vi "Merge Label String.vi"(4 "Draw Major Tick?":bool, 6 "Draw Major Grid?":bool, 7 "Format String":string, 8 "error in (no error)":errorcluster, 9 "Logarithm?":bool, 10 "Tick Value Array":sgl[](array[numeric]), 11 "Value Pair Cluster":T1) -> (0 "error out":errorcluster, 3 "Tick Cluster Array":T2)   [LabVIEW 2020, in "3D Plot.lvclass"]
uses:
  3D Plot.lvclass
  Tick Array.ctl
  Value Pair Cluster.ctl
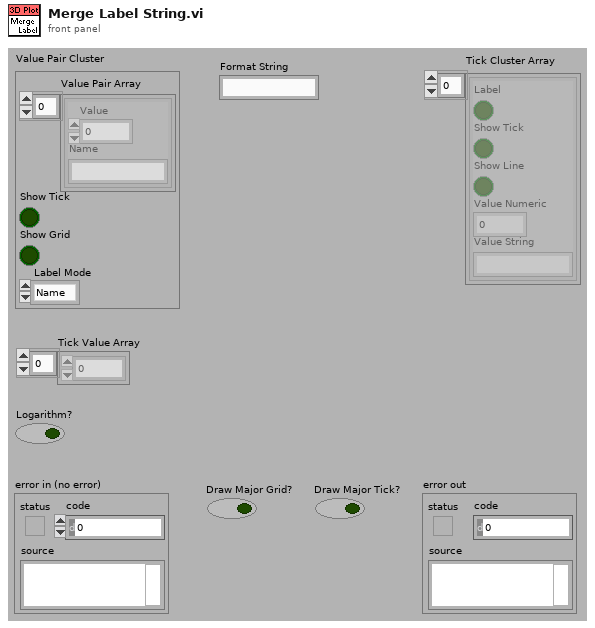
[diagram p1: front panel]
types:
  T1 = typedef "3D Plot.lvclass/Value Pair Cluster.ctl" = cluster{"Value Pair Array":cluster{"Value":sgl, "Name":string}[], "Show Tick":bool, "Show Grid":bool, " Label Mode":enum16{"Name", "Value", "None"}}
  T2 = typedef "3D Plot.lvclass/Tick Array.ctl" = cluster{"Label":bool, "Show Tick":bool, "Show Line":bool, "Value Numeric":sgl, "Value String":string}[]
  T3 = cluster{"Show ticks":bool, "Show ticks":bool, "Show ticks":bool, "Interval":sgl, string}
  T4 = cluster{"Show ticks":bool, "Show ticks":bool, "Show ticks":bool, "Interval":sgl, string}[]
  T5 = cluster{"Show ticks":bool, "Show Tick":bool, "Show Grid":bool, "Value":sgl, "Name":string}
  T6 = cluster{"Show ticks":bool, "Draw Major Tick?":bool, "Draw Major Grid?":bool, "Interval":sgl, string}
  T7 = cluster{"Show ticks":bool, "Show Tick":bool, "Show Grid":bool, "Interval":sgl, "Name":string}
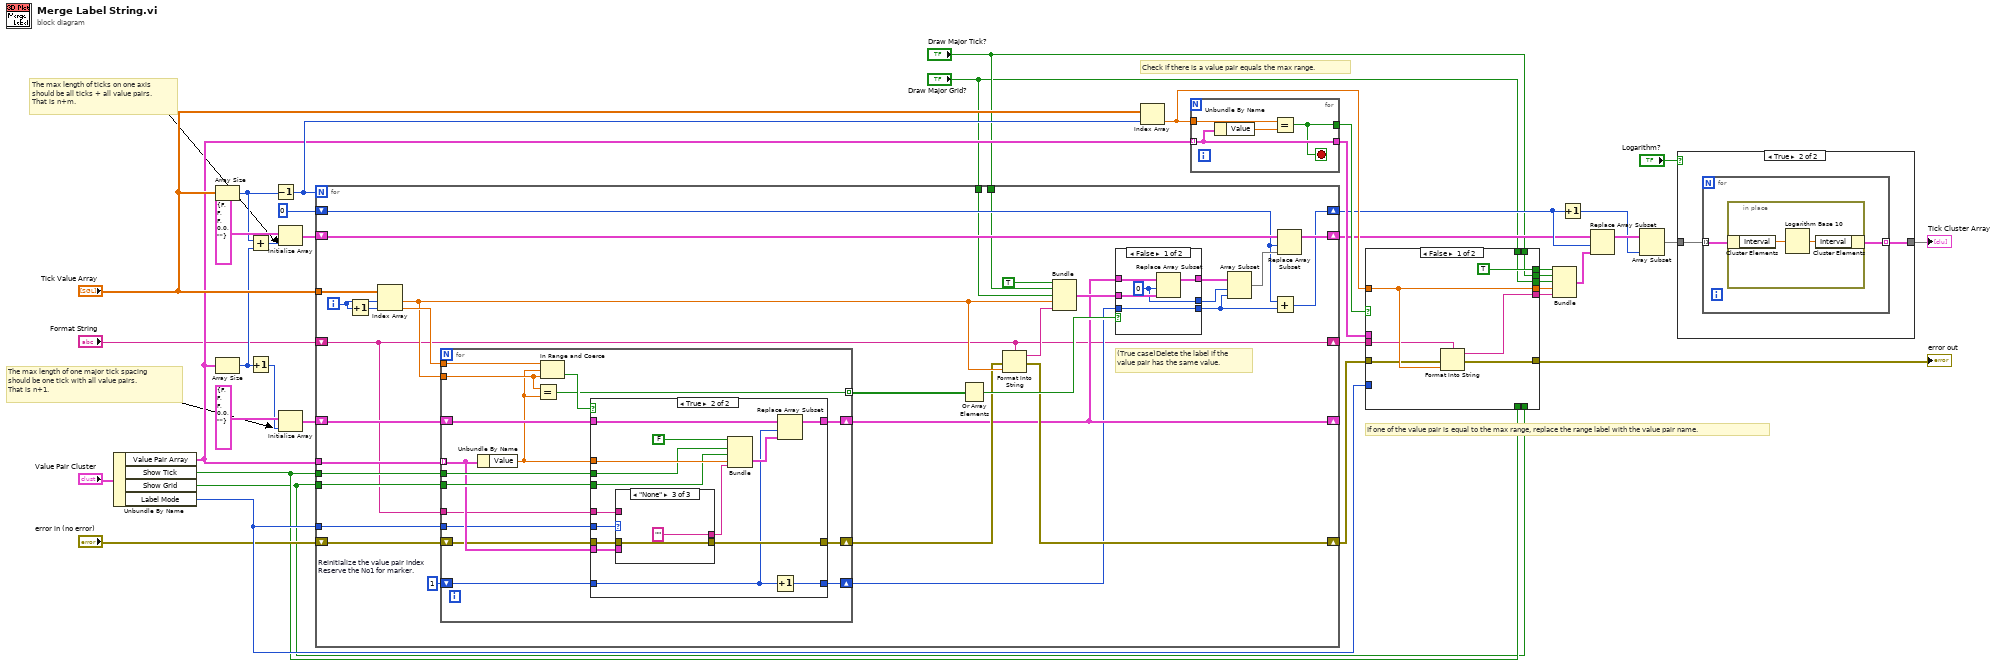
[diagram p0: block diagram]
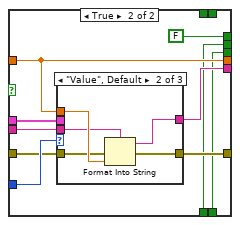
[diagram p3: hidden frame]
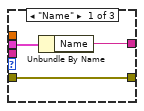
[diagram p4: hidden frame]
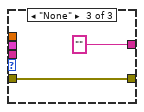
[diagram p5: hidden frame]
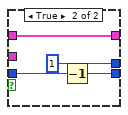
[diagram p6: hidden frame]
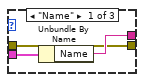
[diagram p8: hidden frame]
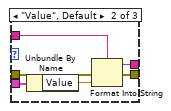
[diagram p9: hidden frame]
diagram:
  # "Check if there is a value pair equals the max range."
  # "The max length of ticks on one axis\nshould be all ticks + all value pairs.\nThat is n+m."
  # "The max length of one major tick spacing \nshould be one tick with all value pairs.\nThat is n+1."
  # "If one of the value pair is equal to the max range, replace the range label with the value pair name."
  n1 = Unbundle By Name("Value Pair Cluster") -> ("Value Pair Array"=w23:cluster{"Value":sgl, "Name":string}[], "Show Tick"=w2:bool, "Show Grid"=w1:bool, "Label Mode"=w34:enum16{"Name", "Value", "None"})
  n2 = Array Size(array="Tick Value Array") -> (size(s)=w19:i32)
  n3 = Array Size(array=w23) -> (size(s)=w18:i32)
  n4 = Add(x=w19, y=w18) -> (x+y=w17:i32)
  n5 = Increment(x=w18) -> (x+1=w22:i32)
  n6 = Decrement(x=w19) -> (x-1=w39:i32)
  n7 = Initialize Array(T3 {"Show ticks"=FALSE, "Show ticks"=FALSE, "Show ticks"=FALSE, "Interval"=0.0, ""}, w17) -> (w20:T4)
  n8 = Initialize Array(T3 {"Show ticks"=FALSE, "Show ticks"=FALSE, "Show ticks"=FALSE, "Interval"=0.0, ""}, w22) -> (w24:T4)
  n9 = for {
    N: w39 -> [_]
    tunnel: "Tick Value Array" -> [w70]
    tunnel: w23 -> [w55]
    tunnel: w2 -> [w64]
    tunnel: w1 -> [w63]
    tunnel: w34 -> [w66]
    shift-right: [w47] -> w10
    shift-left: w20 -> [w48]
    shift-right: [w56] -> w27
    shift-left: "error in (no error)" -> [w58]
    shift-right: [w52] -> _
    shift-left: w24 -> [w53]
    shift-right: [w43] -> w12
    shift-left: 0 -> [w45]
    shift-right: [w42] -> w8
    shift-left: "Format String" -> [w42]
    tunnel: "Draw Major Grid?" -> [w40]
    tunnel: "Draw Major Tick?" -> [w41]
    i -> [w68]
    w54 = 1  # Reinitialize the value pair index Reserve the No1 for marker.
    # "(True case)Delete the label if the \nvalue pair has the same value."
    n10 = Increment(x=w68) -> (x+1=w69:i32)
    n11 = Index Array(array=w70, index #1=w68, index #2=w69) -> (element #1=w60:sgl, element #2=w67:sgl)
    n12 = for {
      tunnel: w55 -> [w88] mode=indexing
      shift-right: [w94] -> w52
      shift-left: w53 -> [w93]
      tunnel: w67 -> [w96]
      tunnel: w60 -> [w89]
      tunnel: w66 -> [w86]
      tunnel: w42 -> [w87]
      tunnel: [w90] -> w62 mode=indexing
      tunnel: w64 -> [w92]
      tunnel: w63 -> [w91]
      shift-right: [w84] -> w57
      shift-left: w58 -> [w83]
      shift-right: [w81] -> w49
      shift-left: w54 -> [w82]
      n13 = Unbundle By Name(w88) -> ("Value"=w85:sgl)
      n14 = Equal?(x=w89, y=w85) -> (x = y?=w90:bool)
      n15 = In Range and Coerce(upper limit=w96, x=w85, lower limit=w89) -> (In Range?=w95:bool)  [unwired: 1 out]
      n16 = case shown="True" w95 {
        tunnel: w85 -> [_ w114]
        tunnel: [w99 w103] -> w94
        tunnel: w93 -> [w99 w104]
        tunnel: w92 -> [_ w112]
        tunnel: w91 -> [_ w111]
        tunnel: w88 -> [_ w110]
        tunnel: w87 -> [_ w109]
        tunnel: w86 -> [_ w108]
        tunnel: [w98 w106] -> w84
        tunnel: w83 -> [w98 w105]
        tunnel: w82 -> [w97 w100]
        tunnel: [w97 w101] -> w81
        frame False {
        }
        frame True {
          n17 = case shown="\"None\"" w108 {
            tunnel: w110 -> [w117 w123 _]
            tunnel: [w116 w120 ""] -> w107
            tunnel: w109 -> [_ w122 _]
            tunnel: [w115 w119 w124] -> w106
            tunnel: w105 -> [w115 w118 w124]
            frame "Name" {
              n18 = Unbundle By Name(w117) -> ("Name"=w116:string)
            }
            frame "Value", Default {
              n19 = Unbundle By Name(w123) -> ("Value"=w121:sgl)
              n20 = Format Into String(format string=w122, error in=w118, w121) -> (resulting string=w120:string, error out=w119:errorcluster)  [unwired: 1 in]
            }
            frame "None" {
            }
          }
          n21 = Bundle("Show ticks"=FALSE, "Show Tick"=w112, "Show Grid"=w111, "Value"=w114, "Name"=w107) -> (w102:T5)  [unwired: 1 out]
          n22 = Increment(x=w100) -> (x+1=w101:i32)
          n23 = Replace Array Subset(array=w104, new element=w102, index=w100) -> (w103:T4)
        }
      }
    }
    n24 = Or Array Elements(Boolean array=w62) -> (logical OR=w61:bool)
    n25 = Format Into String(format string=w42, error in=w57, w60) -> (resulting string=w59:string, error out=w56:errorcluster)  [unwired: 1 in]
    n26 = Bundle("Show ticks"=TRUE, "Draw Major Tick?"=w41, "Draw Major Grid?"=w40, "Interval"=w60, w59) -> (w65:T6)  [unwired: 1 out]
    n27 = case shown="False" w61 {
      tunnel: w52 -> [w76 w80]
      tunnel: w65 -> [w75 _]
      tunnel: [w74 w80] -> w51
      tunnel: [w73 1] -> w50
      tunnel: w49 -> [w72 w78]
      tunnel: [w72 w77] -> w44
      frame False {
        w73 = 0 ("index")
        n28 = Replace Array Subset(array=w76, new element=w75, index=w73) -> (w74:T4)
      }
      frame True {
        n29 = Decrement(x=w78) -> (x-1=w77:i32)
      }
    }
    n30 = Array Subset(array=w51, index=w50, length=w44) -> (w46:T4)
    n31 = Add(x=w45, y=w44) -> (x+y=w43:i32)
    n32 = Replace Array Subset(array=w48, new element=w46, index=w45) -> (w47:T4)
  }
  n33 = Index Array(array="Tick Value Array", index=w39) -> (element=w37:sgl)
  n34 = for {
    tunnel: w23 -> [w127] mode=indexing
    tunnel: [w126] -> w38
    tunnel: w37 -> [w128]
    tunnel: [w127] -> w33
    stop <- w126 stop-if-true
    n35 = Unbundle By Name(w127) -> ("Value"=w129:sgl)
    n36 = Equal?(x=w128, y=w129) -> (x = y?=w126:bool)
  }
  n37 = case shown="False" w38 {
    tunnel: w8 -> [w136 w145]
    tunnel: w37 -> [w137 w143]
    tunnel: [w137 w143] -> w36
    tunnel: [w135 w144] -> w35
    tunnel: w34 -> [_ w146]
    tunnel: w33 -> [_ w147]
    tunnel: w27 -> [w133 w142]
    tunnel: [w134 w141] -> w26
    tunnel: [TRUE ("Show ticks") FALSE ("Show ticks")] -> w7
    tunnel: [w131 w139] -> w6
    tunnel: "Draw Major Tick?" -> [w131 _]
    tunnel: [w130 w138] -> w4
    tunnel: "Draw Major Grid?" -> [w130 _]
    tunnel: w2 -> [_ w139]
    tunnel: w1 -> [_ w138]
    frame False {
      n38 = Format Into String(format string=w136, error in=w133, w137) -> (resulting string=w135:string, error out=w134:errorcluster)  [unwired: 1 in]
    }
    frame True {
      n39 = case shown="\"Value\", Default" w146 {
        tunnel: w147 -> [w150 _ _]
        tunnel: [w149 w153 ""] -> w144
        tunnel: w145 -> [_ w154 _]
        tunnel: w143 -> [_ w155 _]
        tunnel: w142 -> [w148 w152 w156]
        tunnel: [w148 w151 w156] -> w141
        frame "Name" {
          n40 = Unbundle By Name(w150) -> ("Name"=w149:string)
        }
        frame "Value", Default {
          n41 = Format Into String(format string=w154, error in=w152, w155) -> (resulting string=w153:string, error out=w151:errorcluster)  [unwired: 1 in]
        }
        frame "None" {
        }
      }
    }
  }
  "error out" <- w26
  n42 = Bundle("Show ticks"=w7, "Show Tick"=w6, "Show Grid"=w4, "Interval"=w36, "Name"=w35) -> (w15:T7)  [unwired: 1 out]
  n43 = Increment(x=w12) -> (x+1=w11:i32)
  n44 = Replace Array Subset(array=w10, new element=w15, index=w12) -> (w14:T4)
  n45 = Array Subset(array=w14, length=w11) -> (w13:T4)  [unwired: 1 in]
  n46 = case shown="True" "Logarithm?" {
    tunnel: w13 -> [w158 w160]
    tunnel: [w158 w159] -> w29
    frame False {
    }
    frame True {
      n47 = for {
        tunnel: w160 -> [w162] mode=indexing
        tunnel: [w161] -> w159 mode=indexing
        n48 = in-place {
          n49 = in-place-cluster #1(w162) -> ("Interval"=w164:sgl)
          n50 = Logarithm Base 10(1:w164) -> (0:w163:sgl)
          n51 = in-place-cluster #1("Interval"=w163) -> (w161:T3)
        }
      }
    }
  }
  "Tick Cluster Array" <- w29
